vi "Initialize Light Stack.vi"(8 "error in":errorcluster, 11 "PLC in":refnum<class "PLC.lvclass">) -> (0 "error out":errorcluster, 3 "PLC out":refnum<class "PLC.lvclass">)   [LabVIEW 2018, in "PLC.lvlib" / "PLC.lvclass"]
uses:
  PLC.lvclass
  PLC.lvclass/PLC.ctl
  PPLs/PLC/Light Stack/Light Stack.lvlibp/Light Stack.lvclass
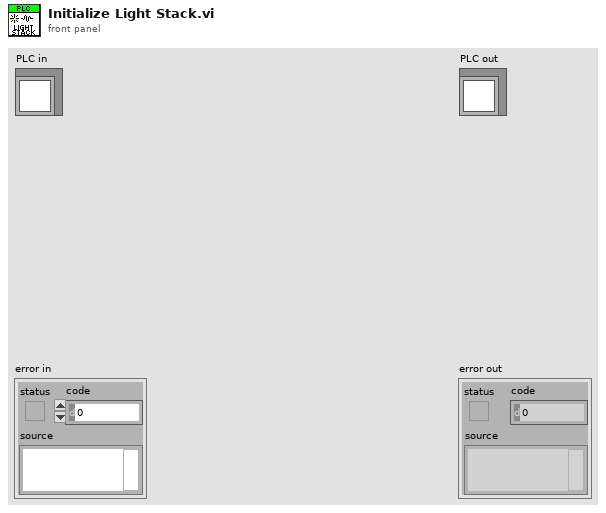
[diagram p1: front panel]
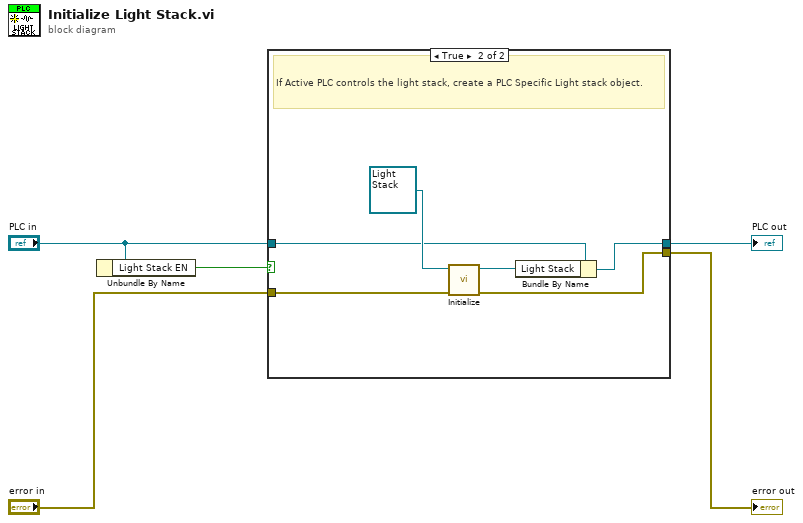
[diagram p0: block diagram]
diagram:
  n1 = Unbundle By Name("PLC in") -> ("Light Stack EN"=w3:bool)
  n2 = case shown="True" w3 {
    tunnel: "PLC in" -> [w7 w11]
    tunnel: "error in" -> [w6 w13]
    tunnel: [w7 w10] -> w5
    tunnel: [w6 w8] -> w4
    frame False {
      # "If this PLC does not control the light stack, do nothing"
    }
    frame True {
      # "If Active PLC controls the light stack, create a PLC Specific Light stack object."
      n3 = call "Initialize.vi"("error in"=w13, "Light Stack in"=refnum<class "Light Stack.lvclass"> refnum) -> ("error out"=w8:errorcluster, "Light Stack out"=w9:refnum<class "Light Stack.lvclass">)  [unwired: 8 in]
      n4 = Bundle By Name(cluster=w11, "Light Stack"=w9) -> (w10:refnum<class "PLC.lvclass">)
    }
  }
  "error out" <- w4
  "PLC out" <- w5
